vi "Memory.Pointer.Copy.vi"   [LabVIEW 2016, in "Memory Manager.lvlib" / "Memory.Pointer.lvclass"]
uses:
  Memory.Pointer.lvclass
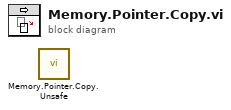
[diagram p0: block diagram]
diagram:
  n1 = call "Memory.Pointer.Copy.Unsafe.vi"() -> ()  [unwired: 8 in, 4 out]
